vi "LuaVIEW Poll Print Buffer.vi"(5 "LuaVIEW reference in":T1, 7 "read all?":bool, 9 "read index in":i32, 11 "error in (no error)":errorcluster) -> (4 "text":string, 6 "LuaVIEW reference out":T1, 8 "text gap?":bool, 10 "read index out":i32, 15 "error out":errorcluster)   [LabVIEW 2012]
doc: "Each LuaVIEW state is provided with a private print buffer. Using the lv.print() function, text can be printed to this buffer on a per-script or per-task basis. This VI allows polling of the content of these print buffers for display purposes. One option is to empty the entire content, and display that. This limits the amount of displayed text to the size of the circular print buffer (32768 characters). Alternatively, the read index can be used to return only the newly printed text, if any. By frequently polling the buffer and appending the returned text to previously read text, you can display more text than fits inside the buffer.\n\nThis VI is exceptional because it is designed to poll the print buffer of a LuaVIEW state while other operations on that state are ongoing: normally actions on the same LuaVIEW state must be serialized. This implies that it can be used inside a loop that is asynchronous from the script or task execution."
uses:
  typedefs/t_LuaVIEW Reference.ctl
  typedefs/t_LuaVIEW CIN Spinlocked Actions.ctl
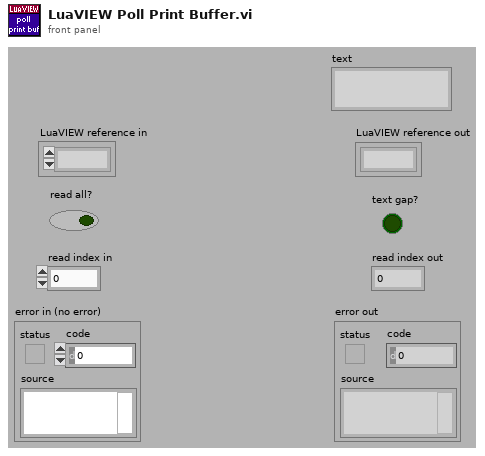
[diagram p1: front panel]
types:
  T1 = typedef "t_LuaVIEW Reference.ctl" = refnum<k1>
  T2 = typedef "t_LuaVIEW CIN Spinlocked Actions.ctl" = enum16{"totals", "taskcount", "open", "registerpublic", "registerexport", "revokeexports", "unregnextpublic", "usepublic", "pollexport", "close", "startyieldtest", "endyieldtest", "pollprintbuffer"}
  T3 = typedef "et_LuaVIEW CIN Results.ctl" = enum16{"OK", "error", "main", "call", "clonecall", "modulecall", "exportcall", "index", "yield"}
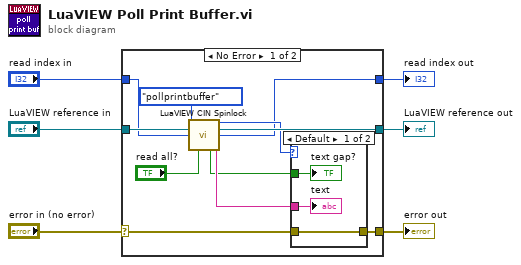
[diagram p0: block diagram]
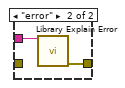
[diagram p2: hidden frame]
diagram:
  n1 = case shown="No Error" "error in (no error)" {
    selector: "error in (no error)" -> [w12 w25]
    tunnel: [w16 w24] -> w6
    tunnel: [w15 w25] -> w5
    tunnel: "LuaVIEW reference in" -> [w17 w24]
    tunnel: "read index in" -> [w9 w23]
    tunnel: [w8 w23] -> w1
    frame No Error {
      n2 = call "LuaVIEW CIN Spinlock.vi"("action"=t_LuaVIEW_CIN_Spinlocked_Actions."pollprintbuffer", "LuaVIEW reference in"=w17, "index in"=w9, "boolean in"="read all?") -> ("result"=w14:T3, "LuaVIEW reference out"=w16:T1, "index out"=w8:i32, "boolean out"=w7:bool, "string out"=w13:string)  [unwired: 5 in, 2 out]
      n3 = case shown="Default" w14 {
        tunnel: w13 -> [w19 w22]
        tunnel: [w20 w21] -> w15
        tunnel: w12 -> [w20 _]
        tunnel: w7 -> [w18 _]
        frame Default {
          "text" <- w19
          "text gap?" <- w18
        }
        frame "error" {
          n4 = call "Library Explain Error.vi"("explanation prefix (none)"=w22) -> ("explained error"=w21:errorcluster)  [unwired: 14 in]
        }
      }
    }
    frame Error {
    }
  }
  "LuaVIEW reference out" <- w6
  "error out" <- w5
  "read index out" <- w1
